vi "Update Header.vi"(11 "CIFFIFO in":refnum<class "CIFfifo.lvclass">) -> (3 "CIFFIFO out":refnum<class "CIFfifo.lvclass">)   [LabVIEW 2021, in "CIFfifo.lvclass"]
uses:
  CIFfifo.lvclass
  CIFfifo.lvclass/CIFfifo.ctl
  <vilib>/CIF Foundation/CIF Utilities/Time/System Time/LabVIEW Time to TAI Time.vi
  <vilib>/CIF Foundation/CIF Utilities/Time/Time_CIF_U.lvlib
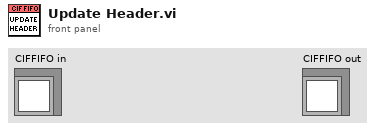
[diagram p1: front panel]
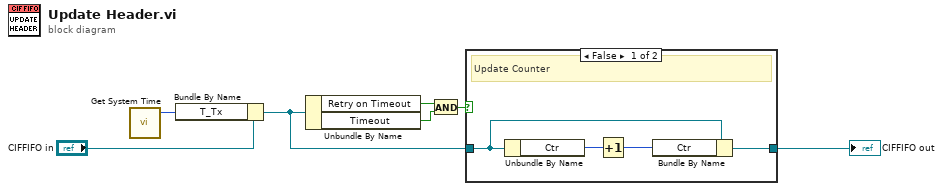
[diagram p0: block diagram]
diagram:
  n1 = call <vilib>:"Get System Time.vi"() -> ("Time (ns)"=w1:i64)  [unwired: 5 in]
  n2 = Bundle By Name(cluster="CIFFIFO in", "T_Tx"=w1) -> (w2:refnum<class "CIFfifo.lvclass">)
  n3 = Unbundle By Name(w2) -> ("Retry on Timeout"=w5:bool, "Timeout"=w4:bool)
  n4 = And(x=w5, y=w4) -> (x .and. y?=w3:bool)
  n5 = case shown="False" w3 {
    tunnel: w2 -> [w11 w12]
    tunnel: [w10 w12] -> w6
    frame False {
      # "Update Counter"
      n6 = Unbundle By Name(w11) -> ("Ctr"=w9:u64)
      n7 = Increment(x=w9) -> (x+1=w8:u64)
      n8 = Bundle By Name(cluster=w11, "Ctr"=w8) -> (w10:refnum<class "CIFfifo.lvclass">)
    }
    frame True {
      # "Retry last packet"
    }
  }
  "CIFFIFO out" <- w6
